vi "Apply EQ coeff to wideband data.vi"() -> ()   [LabVIEW 2019]
uses:
  SubVIs/Low-level/TypeDefs/Constants.ctl
  SubVIs/Low-level/Utility/Global Constants.vi
panel:
  out "EQ FIR  time":dbl format="%#_6p"
  in  "Max FIR gain":dbl=6.0 format="%#_13g"
  out "Magnitude response":cluster{"Ramp Pattern":dbl[], dbl[]}[](graph) caption="XY Graph - Dark"
  in  "Channel response":path=path "C:/ProgramData/Noffz/coeff.bin"
  in  "repeat signal":i32=1
  out "FIR coeff":dbl[][](graph)
  in  "FIR taps":i32=32
  out "IQ signals":dbl[][](graph)
  out "EQ spectrum time":dbl format="%#_6p"
  out "Signal amplitude":dbl[][](graph)
  in  "data":path=path "C:/Barkhausen mmWave radar/Analysis data/1GBW_upper.dat"
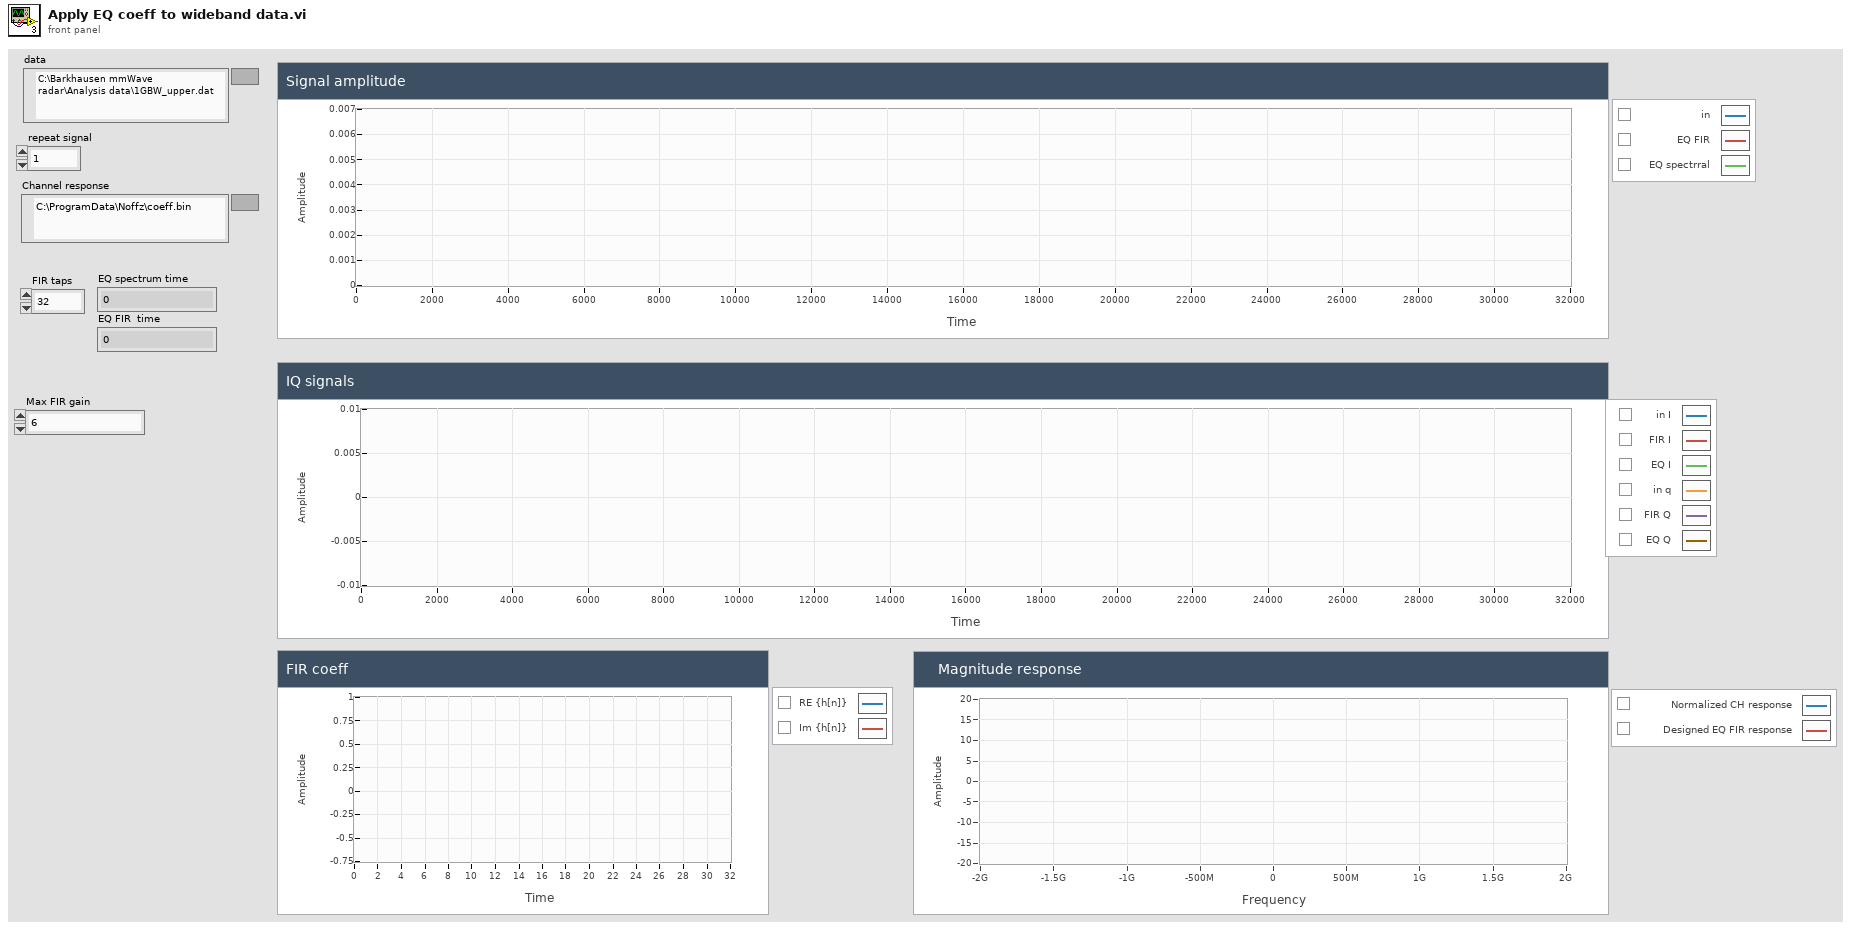
[diagram p1: front panel]
types:
  T1 = cluster{"frequency offset (Hz)":dbl[], "response":cdb[]}
  T2 = typedef "Constants.ctl" = cluster{"data clock rate (Hz)":dbl, "sample rate (Hz)":dbl, "sample rate selector string":string, "default tx bitfile path":path, "default rx bitfile path":path, "default proc bitfile path":path}
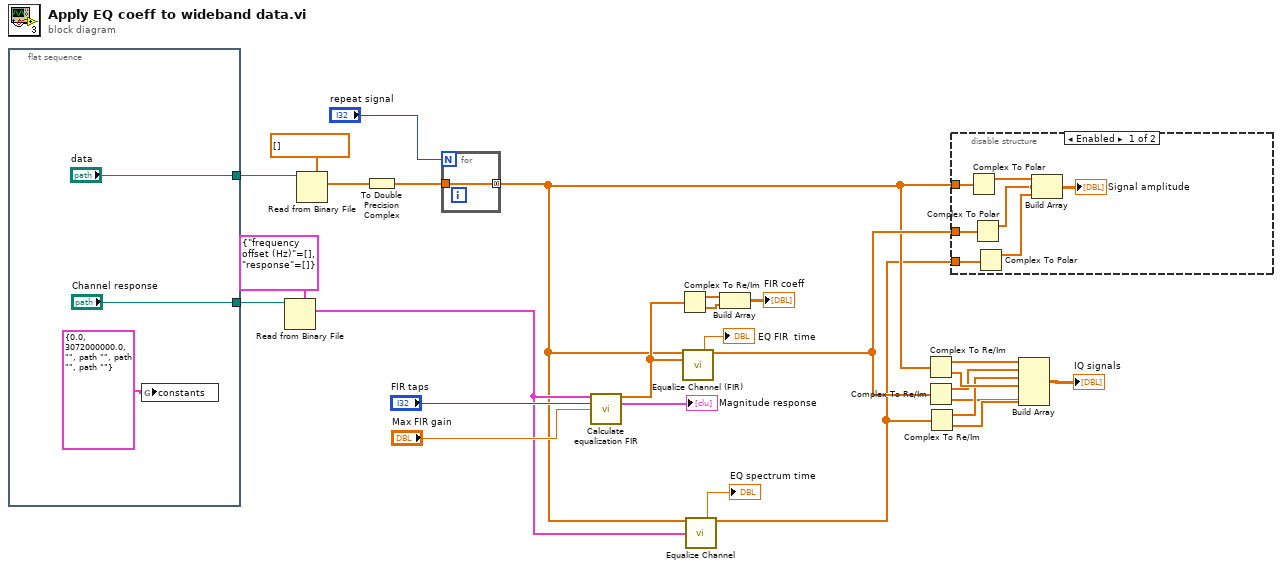
[diagram p0: block diagram]
diagram:
  n1 = flat-sequence {
    tunnel: ["data"] -> w27
    tunnel: ["Channel response"] -> w24
    frame #0 {
      n2 = global write "Global Constants.vi" "constants"(T2 {"data clock rate (Hz)"=0.0, "sample rate (Hz)"=3072000000.0, "sample rate selector string"="", "default tx bitfile path"=path "", "default rx bitfile path"=path "", "default proc bitfile path"=path ""} ("constants")) -> ()
    }
  }
  n3 = Read from Binary File(5:T1 {"frequency offset (Hz)"=[], "response"=[]} ("channel"), 11:w24) -> (2:w11:T1)  [unwired: 4 in, 3 out]
  n4 = Read from Binary File(5:csg[] [], 11:w27) -> (2:w23:csg[])  [unwired: 4 in, 3 out]
  n5 = To Double Precision Complex(1:w23) -> (0:w21:cdb[])
  n6 = for {
    N: "repeat signal" -> [_]
    tunnel: w21 -> [w31]
    tunnel: [w31] -> w4 mode=concatenating
  }
  n7 = call "Calculate equalization FIR.vi"("channel"=w11, "FIR taps"="FIR taps", "Max FIR gain"="Max FIR gain") -> ("EQ FIR coeff"=w10:cdb[], "Mag response"=→"Magnitude response":cluster{"xi used":dbl[], "yi":dbl[]}[])  [unwired: 10 in, 1 out]
  n8 = Complex To Re/Im(x + iy=w10) -> (x=w16:dbl[], y=w15:dbl[])
  n9 = call "Equalize Channel (FIR).vi"("input data"=w4, "FIR coeff"=w10) -> ("processing time"=→"EQ FIR  time":dbl, "output data"=w7:cdb[])  [unwired: 12 in]
  n10 = call "Equalize Channel.vi"("input data"=w4, "channel"=w11) -> ("processing duration"=→"EQ spectrum time":dbl, "output data"=w3:cdb[])  [unwired: 12 in]
  n11 = Build Array(w16, w15) -> (→"FIR coeff":dbl[][])
  n12 = Complex To Re/Im(x + iy=w4) -> (x=w19:dbl[], y=w18:dbl[])
  n13 = Complex To Re/Im(x + iy=w7) -> (x=w6:dbl[], y=w5:dbl[])
  n14 = Complex To Re/Im(x + iy=w3) -> (x=w8:dbl[], y=w17:dbl[])
  n15 = disable-structure shown="Enabled" {
    disable-tunnel: w4 -> [w37 _]
    disable-tunnel: w7 -> [w35 _]
    disable-tunnel: w3 -> [w34 _]
    frame Enabled {
      n16 = Complex To Polar(r * e^(i*theta)=w37) -> (r=w36:dbl[])  [unwired: 1 out]
      n17 = Complex To Polar(r * e^(i*theta)=w35) -> (r=w33:dbl[])  [unwired: 1 out]
      n18 = Complex To Polar(r * e^(i*theta)=w34) -> (r=w32:dbl[])  [unwired: 1 out]
      n19 = Build Array(w36, w33, w32) -> (→"Signal amplitude":dbl[][])
    }
    frame Disabled {
    }
  }
  n20 = Build Array(w19, w6, w8, w18, w5, w17) -> (→"IQ signals":dbl[][])
